vi "get_settings_cluster.vi"(8 "error in (no error)":errorcluster, 11 "GenericPlugin in":refnum<class "TrajectoryCN090716SpiralScan.lvclass">) -> (0 "error out":errorcluster, 2 "settings cluster":variant, 3 "GenericPlugin out":refnum<class "TrajectoryCN090716SpiralScan.lvclass">)   [LabVIEW 2010, in "TrajectoryCN090716SpiralScan.lvclass"]
uses:
  TrajectoryCN090716SpiralScan.lvclass
  TrajectoryCN090716SpiralScan.lvclass/TrajectoryCN090716SpiralScan.ctl
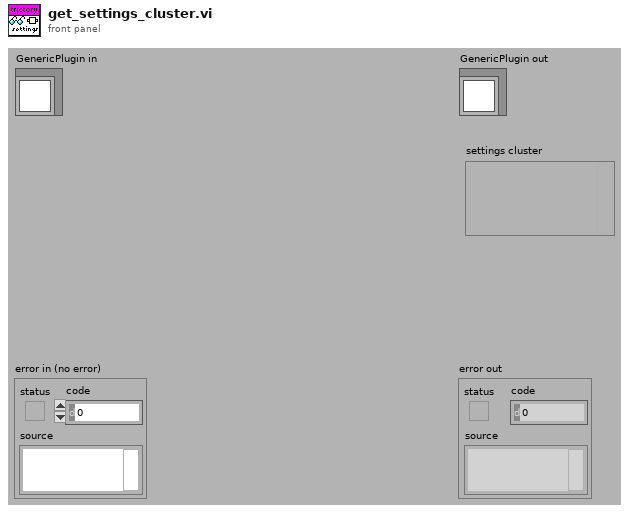
[diagram p1: front panel]
types:
  T1 = typedef "TrajectoryCN090716SpiralScan.lvclass/settings_cluster.ctl" = cluster{"z-motion":enum16{"Sine", "Saw-tooth"}, "spirals":i32, "turns per spiral":i32, "pixels per turn":i32, "z amplitude":dbl[unit], "spiral amplitude":dbl[unit], "circularity":dbl, "phase correction":dbl[unit], "amplitude correction factor":dbl}
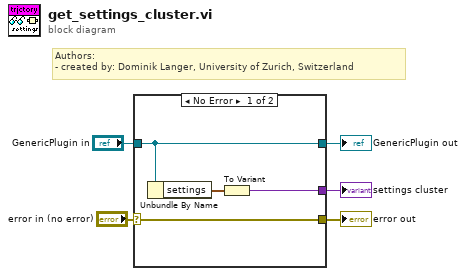
[diagram p0: block diagram]
diagram:
  # "Authors: \n- created by: Dominik Langer, University of Zurich, Switzerland"
  n1 = case shown="No Error" "error in (no error)" {
    selector: "error in (no error)" -> [w7 w11]
    tunnel: [w8 _] -> w5
    tunnel: "GenericPlugin in" -> [w6 w10]
    tunnel: [w7 w11] -> w2
    tunnel: [w6 w10] -> w1
    frame No Error {
      n2 = Unbundle By Name(w6) -> ("settings"=w9:T1)
      n3 = To Variant(anything=w9) -> (Variant=w8:variant)
    }
    frame Error {
    }
  }
  "error out" <- w2
  "GenericPlugin out" <- w1
  "settings cluster" <- w5
